vi "Decimal Hours.vi"() -> (0 "decimal hours now":dbl format="%.5f")   [LabVIEW 2019]
doc: "This VI returns the decimal hour equivalent of the current time. For instance, if it is now 3:45 PM, 'decimal hours now' equals 15.75.\n\nResolution is 1 ms, or whatever the limitation of this implementation of LabVIEW might be.\n\nTime overflows after 2^32 ms, which is 50 days."
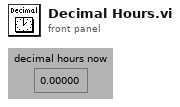
[diagram p1: front panel]
types:
  T1 = cluster{"second":i32, "minute":i32, "hour":i32, "day of month":i32, "month":i32, "year":i32, "day of week":i32, "day of year":i32, "is DST":i32}
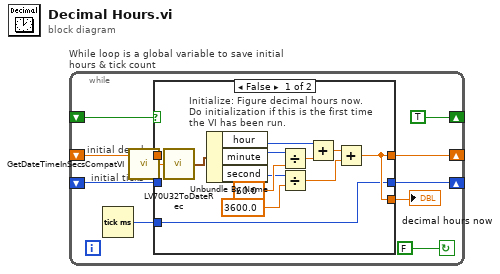
[diagram p0: block diagram]
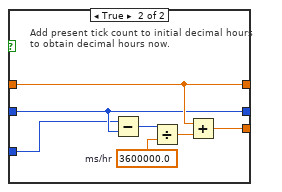
[diagram p2: hidden frame]
diagram:
  n1 = while "While loop is a global variable to save initial hours & tick count" {
    shift-left: _ -> [w9]
    shift-right: [w8] -> _
    shift-left: _ -> [w3]
    shift-right: [TRUE] -> _
    shift-left: _ -> [w6]
    shift-right: [w7] -> _
    stop <- FALSE continue-if-true
    # "initial dec. hrs"
    # "initial ticks"
    n2 = Tick Count (ms)() -> (millisecond timer value=w2:u32)
    n3 = case shown="False" w3 {
      tunnel: [w16 w25] -> w4
      tunnel: w6 -> [_ w24]
      tunnel: [w11 w24] -> w7
      tunnel: w9 -> [_ w26]
      tunnel: [w16 w26] -> w8
      tunnel: w2 -> [w11 w22]
      frame False {
        # "Initialize: Figure decimal hours now.\nDo initialization if this is the first time\nthe VI has been run."
        n4 = call <vilib>:"GetDateTimeInSecsCompatVI.vi"() -> ("double precision float"=w10:dbl)  [unwired: 1 in]
        n5 = call <vilib>:"LV70U32ToDateRec.vi"("Time"=w10) -> ("date time rec"=w15:T1)
        n6 = Unbundle By Name(w15) -> ("hour"=w14:i32, "minute"=w13:i32, "second"=w12:i32)
        n7 = Divide(x=w13, y=60.0) -> (x/y=w19:dbl)
        n8 = Divide(x=w12, y=3600.0) -> (x/y=w20:dbl)
        n9 = Add(x=w14, y=w19) -> (x+y=w21:dbl)
        n10 = Add(x=w21, y=w20) -> (x+y=w16:dbl)
      }
      frame True {
        w28 = 3600000.0  # ms/hr
        # "Add present tick count to initial decimal hours\nto obtain decimal hours now."
        n11 = Subtract(x=w22, y=w24) -> (x-y=w23:u32)
        n12 = Divide(x=w23, y=w28) -> (x/y=w27:dbl)
        n13 = Add(x=w26, y=w27) -> (x+y=w25:dbl)
      }
    }
    "decimal hours now" <- w4
  }
